vi "McAfee Poke Test.vi"() -> ()   [LabVIEW 2015]
panel:
  out "FPA":bool
  out "McAfee":dbl format="%.1f%%"
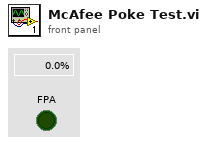
[diagram p1: front panel]
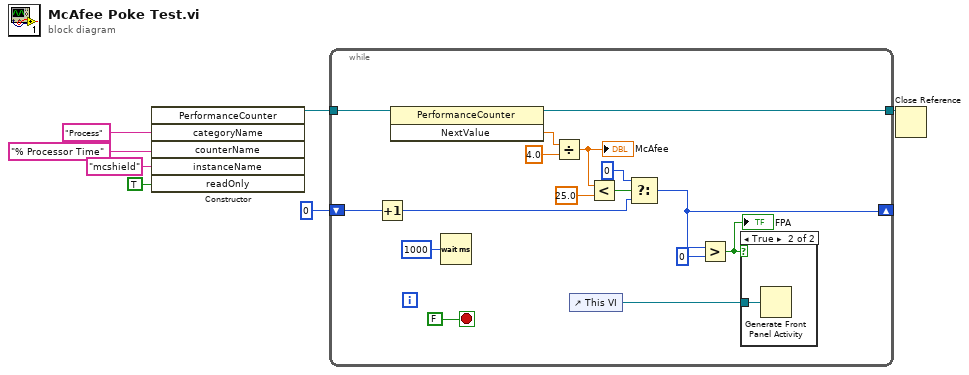
[diagram p0: block diagram]
diagram:
  n1 = constructor class="PerformanceCounter"("categoryName"="Process", "counterName"="% Processor Time", "instanceName"="mcshield", "readOnly"=TRUE) -> (reference out=w3:refnum<k24>)  [unwired: 3 in, 6 out]
  n2 = while {
    tunnel: w3 -> [w22]
    tunnel: [w21] -> w2
    shift-right: [w12] -> _
    shift-left: 0 -> [w15]
    stop <- FALSE stop-if-true
    n3 = Increment(x=w15) -> (x+1=w14:i32)
    n4 = invoke class="PerformanceCounter" method="NextValue"(reference=w22) -> (reference out=w21:refnum<k24>, "NextValue"=w20:sgl)  [unwired: 2 in, 1 out]
    n5 = Wait (ms)(milliseconds to wait=u32 1000) -> ()  [unwired: 1 out]
    n6 = Divide(x=w20, y=sgl 4.0) -> (x/y=w18:sgl)
    "McAfee" <- w18
    n7 = control-ref of="This VI"() -> (w9:refnum<vi>)
    n8 = Less?(x=w18, y=sgl 25.0) -> (x < y?=w16:bool)
    n9 = Select(t=0, s=w16, f=w14) -> (s? t:f=w12:i32)
    n10 = Greater?(x=w12, y=0) -> (0:w8:bool)
    "FPA" <- w8
    n11 = case shown="True" w8 {
      tunnel: w9 -> [_ w24]
      frame False {
      }
      frame True {
        n12 = Generate Front Panel Activity(w24) -> ()
      }
    }
  }
  n13 = Close Reference(reference=w2) -> ()  [unwired: 1 in, 1 out]
